vi "RichToFlatnidaqmx_grpc_WriteDigitalLinesRequest.vi"(5 "OutputClusterType":T1, 11 "InputCluster":T4) -> (3 "OutputCluster":T1)   [LabVIEW 2021, in "NI DAQmx_server.lvlib"]
uses:
  NI DAQmx_server.lvlib
  nidaqmx_grpc_WriteDigitalLinesRequest.ctl
  nidevice_grpc_Session_session/nidevice_grpc_Session_session.lvclass
  nidaqmx_grpc_WriteDigitalLinesRequest_data_layout_enum/nidaqmx_grpc_WriteDigitalLinesRequest_data_layout_enum.lvclass
  nidevice_grpc_Session.ctl
  nidaqmx_grpc_WriteDigitalLinesRequest_Flat.ctl
  nidevice_grpc_Session_Flat.ctl
  nidaqmx_grpc_GroupBy.ctl
  nidevice_grpc_Session_session/nidevice_grpc_Session_session.lvclass/nidevice_grpc_Session_session.ctl
  nidaqmx_grpc_WriteDigitalLinesRequest_data_layout_enum/nidaqmx_grpc_WriteDigitalLinesRequest_data_layout_enum.lvclass/nidaqmx_grpc_WriteDigitalLinesRequest_data_layout_enum.ctl
  nidevice_grpc_Session_session/Getname.vi
  nidevice_grpc_Session_session/Getid.vi
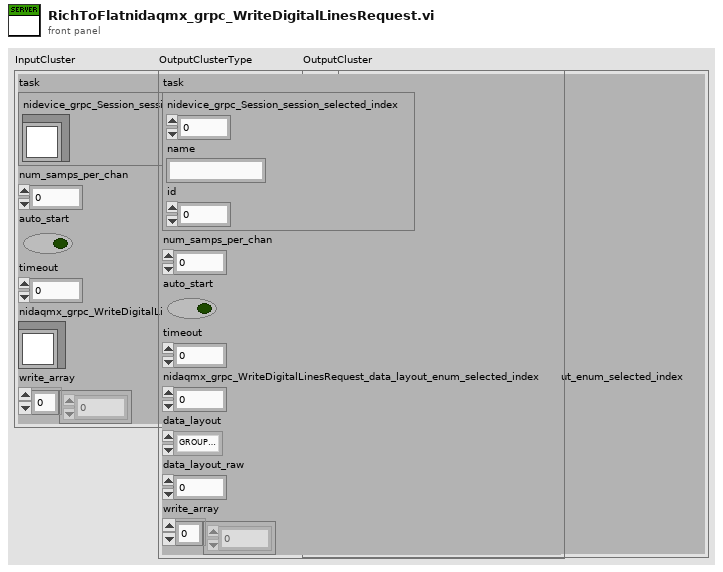
[diagram p1: front panel]
types:
  T1 = typedef "NI DAQmx_server.lvlib/nidaqmx_grpc_WriteDigitalLinesRequest_Flat.ctl" = cluster{"task":T2, "num_samps_per_chan":i32, "auto_start":bool, "timeout":dbl, "nidaqmx_grpc_WriteDigitalLinesRequest_data_layout_enum_selected_index":i32, "data_layout":T3, "data_layout_raw":i32, "write_array":u8[]}
  T2 = typedef "NI DAQmx_server.lvlib/nidevice_grpc_Session_Flat.ctl" = cluster{"nidevice_grpc_Session_session_selected_index":i32, "name":string, "id":u32}
  T3 = typedef "NI DAQmx_server.lvlib/nidaqmx_grpc_GroupBy.ctl" = enum32{"GROUP_BY_GROUP_BY_CHANNEL", "GROUP_BY_GROUP_BY_SCAN_NUMBER"}
  T4 = typedef "NI DAQmx_server.lvlib/nidaqmx_grpc_WriteDigitalLinesRequest.ctl" = cluster{"task":T5, "num_samps_per_chan":i32, "auto_start":bool, "timeout":dbl, "nidaqmx_grpc_WriteDigitalLinesRequest_data_layout_enum":refnum<class "nidaqmx_grpc_WriteDigitalLinesRequest_data_layout_enum.lvclass">, "write_array":u8[]}
  T5 = typedef "NI DAQmx_server.lvlib/nidevice_grpc_Session.ctl" = cluster{"nidevice_grpc_Session_session":refnum<class "nidevice_grpc_Session_session.lvclass">}
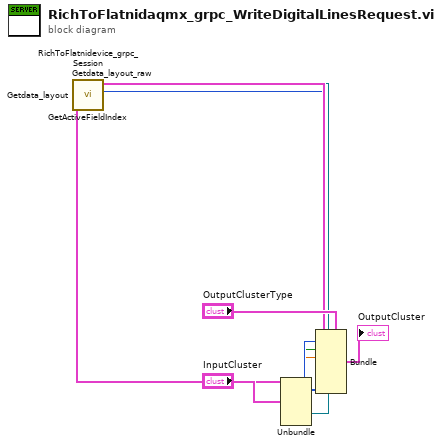
[diagram p0: block diagram]
diagram:
  n1 = Unbundle "Unbundle"("InputCluster") -> ("task"=w10:T5, "num_samps_per_chan"=w8:i32, "auto_start"=w7:bool, "timeout"=w6:dbl, "nidaqmx_grpc_WriteDigitalLinesRequest_data_layout_enum"=w5:refnum<class "nidaqmx_grpc_WriteDigitalLinesRequest_data_layout_enum.lvclass">, "write_array"=w1:u8[])
  n2 = call "Getdata_layout_raw.vi"("OneOfTemplate in"=w5) -> ("Get_Val"=w2:i32)  [unwired: 8 in, 2 out]
  n3 = call "Getdata_layout.vi"("OneOfTemplate in"=w5) -> ("Get_Val"=w3:T3)  [unwired: 8 in, 2 out]
  n4 = call "GetActiveFieldIndex.vi"("OneOfTemplate in"=w5) -> ("Active Field Index"=w4:i32)  [unwired: 8 in, 2 out]
  n5 = call "RichToFlatnidevice_grpc_Session.vi"("InputCluster"=w10) -> ("OutputCluster"=w9:T2)  [unwired: 10 in]
  n6 = Bundle "Bundle"(cluster="OutputClusterType", "task"=w9, "num_samps_per_chan"=w8, "auto_start"=w7, "timeout"=w6, "nidaqmx_grpc_WriteDigitalLinesRequest_data_layout_enum_selected_index"=w4, "data_layout"=w3, "data_layout_raw"=w2, "write_array"=w1) -> (→"OutputCluster":T1)
